vi "Read ModuleHeight.vi"(8 "error in (no error)":errorcluster, 11 "Linear Barcode in":refnum<class "Linear Barcode.lvclass">) -> (0 "error out":errorcluster, 2 "ModuleHeight":u8=1, 3 "Linear Barcode out":refnum<class "Linear Barcode.lvclass">)   [LabVIEW 2013, in "BarCodes.lvlib" / "Linear Barcode.lvclass"]
uses:
  Linear Barcode.lvclass
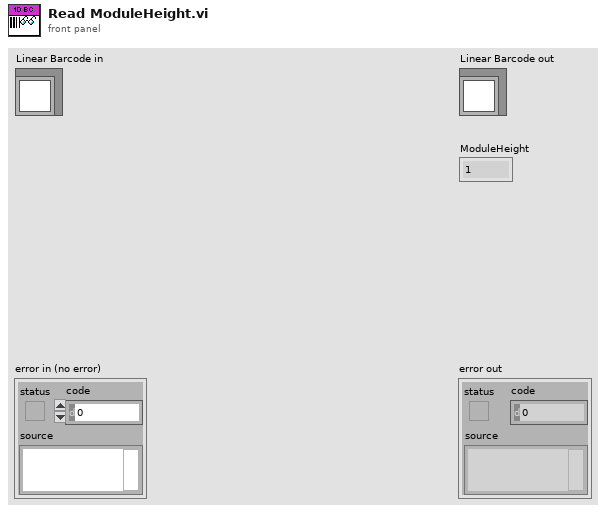
[diagram p1: front panel]
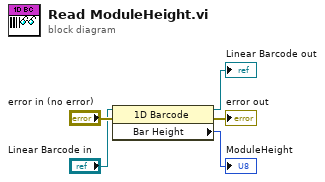
[diagram p0: block diagram]
diagram:
  n1 = property class="1D Barcode"(reference="Linear Barcode in", error in="error in (no error)") -> (reference out=→"Linear Barcode out":refnum<class "Linear Barcode.lvclass">, error out=→"error out":errorcluster, "Bar Height"=→"ModuleHeight":u8)
